vi "get VIPM version string.vi"() -> (3 "version string":string)   [LabVIEW 2010]
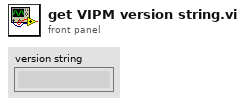
[diagram p1: front panel]
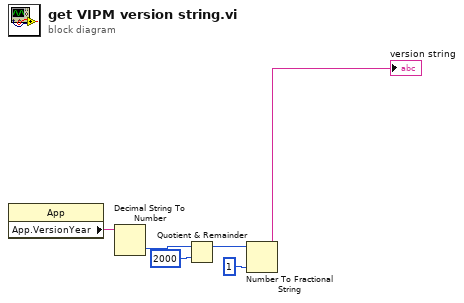
[diagram p0: block diagram]
diagram:
  n1 = property class="App"() -> ("App.VersionYear"=w1:string)  [unwired: 2 in, 2 out]
  n2 = Decimal String To Number(string=w1) -> (number=w2:i32)  [unwired: 2 in, 1 out]
  n3 = Quotient & Remainder(x=w2, y=2000) -> (x-y*floor(x/y)=w4:i32)  [unwired: 1 out]
  n4 = Number To Fractional String(number=w4, precision (6)=i16 1) -> (F-format string=→"version string":string)  [unwired: 2 in]
